vi "Forward Kinematics.vi"(8 "j3":dbl, 9 "j2":dbl, 10 "j1":dbl, 11 "armID":i32) -> (2 "XYZ Out Array":dbl[](array[numeric]))   [LabVIEW 2016]
uses:
  RobotKinematicsDLL.dll
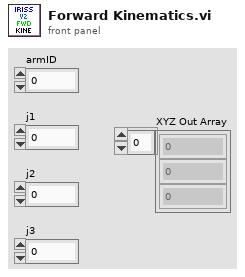
[diagram p1: front panel]
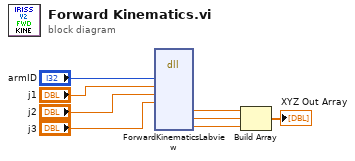
[diagram p0: block diagram]
diagram:
  n1 = dll-call lib="D:/Kevin/IRISS V2 dev/Host Demo/Functions/RobotKinematicsDLL.dll" fn="ForwardKinematicsLabview"("id"="armID", "j1"="j1", "j2"="j2", "j3"="j3") -> ("x"=w4:dbl, "y"=w3:dbl, "z"=w2:dbl)  [unwired: 11 in, 2 out]
  n2 = Build Array(w4, w3, w2) -> (→"XYZ Out Array":dbl[])
